vi "mod_Decimating FIR.vi"(5 "reset":bool, 6 "error in (no error)":errorcluster, 7 "taps":dbl[](array[numeric]), 8 "decimation":i32, 9 "x":dbl[](array[numeric])) -> (0 "error out":errorcluster, 3 "filtered x":dbl[](array[numeric]))   [LabVIEW 2020, in "niAMT.lvlib"]
uses:
  <vilib>/addons/Modulation/niAMT.lvlib
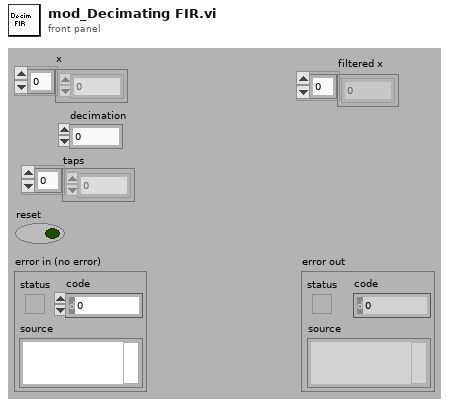
[diagram p1: front panel]
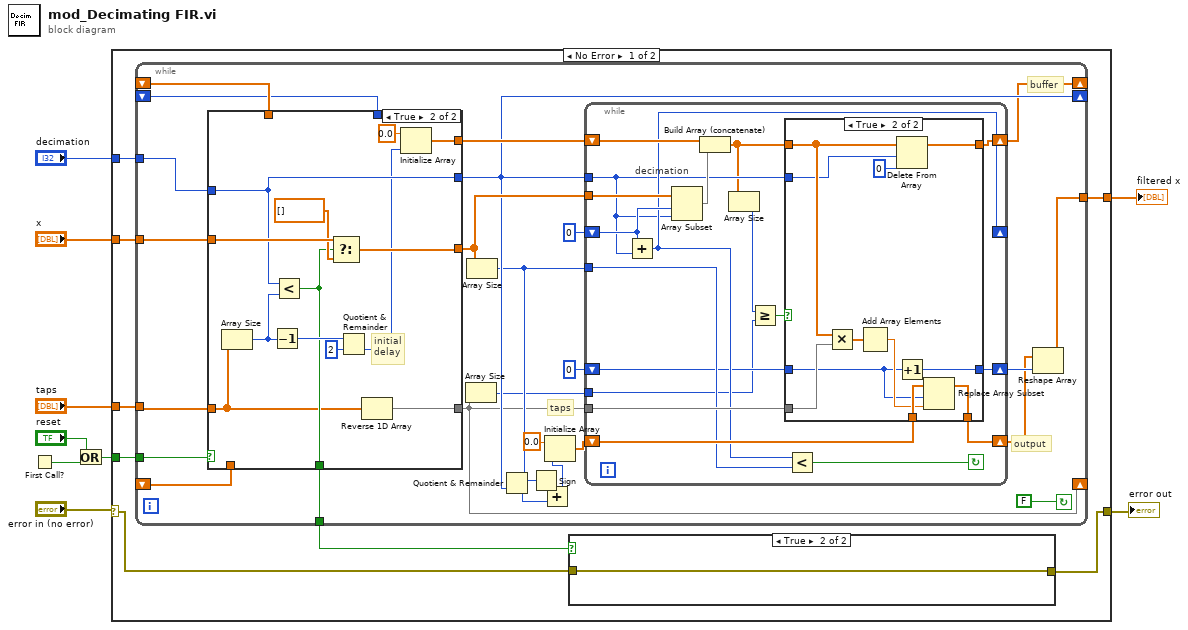
[diagram p0: block diagram]
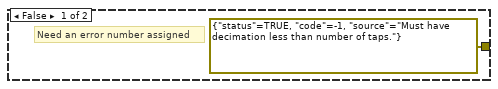
[diagram p2: hidden frame]
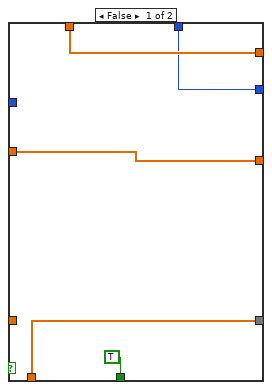
[diagram p4: hidden frame]
diagram:
  n1 = First Call?() -> (First Call?: T/F=w9:bool)
  n2 = Or(x="reset", y=w9) -> (x .or. y?=w5:bool)
  n3 = case shown="No Error" "error in (no error)" {
    selector: "error in (no error)" -> [w11 w98]
    tunnel: "x" -> [w17 w97]
    tunnel: "decimation" -> [w16 _]
    tunnel: "taps" -> [w15 _]
    tunnel: w5 -> [w14 _]
    tunnel: [w10 w98] -> w2
    tunnel: [w13 w97] -> w1
    frame No Error {
      n4 = while {
        tunnel: w14 -> [w45]
        tunnel: w17 -> [w42]
        tunnel: w16 -> [w43]
        tunnel: w15 -> [w24]
        shift-right: [w20] -> _
        shift-left: _ -> [w44]
        shift-right: [w21] -> _
        shift-left: _ -> [w41]
        tunnel: [w29] -> w13
        shift-right: [w26] -> _
        shift-left: _ -> [w40]
        tunnel: [w39] -> w12
        stop <- FALSE continue-if-true
        # "taps"
        # "output"
        # "buffer"
        n5 = case shown="True" w45 {
          tunnel: w24 -> [_ w85]
          tunnel: [w83 w96] -> w20
          tunnel: w44 -> [w83 _]
          tunnel: w43 -> [_ w87]
          tunnel: w42 -> [w82 w92]
          tunnel: [w82 w91] -> w38
          tunnel: [w81 w93] -> w27
          tunnel: w41 -> [w81 _]
          tunnel: [w80 w87] -> w26
          tunnel: w40 -> [w80 _]
          tunnel: [TRUE w89] -> w39
          frame False {
          }
          frame True {
            # "initial\ndelay"
            n6 = Array Size(array=w85) -> (size(s)=w84:i32)
            n7 = Decrement(x=w84) -> (x-1=w94:i32)
            n8 = Less?(x=w87, y=w84) -> (x < y?=w89:bool)
            n9 = Select(t=w92, s=w89, f=dbl[] []) -> (s? t:f=w91:dbl[])
            n10 = Quotient & Remainder(x=w94, y=2) -> (floor(x/y)=w86:i32)  [unwired: 1 out]
            n11 = Reverse 1D Array(array=w85) -> (reversed array=w96:dbl[])
            n12 = Initialize Array(0.0 ("element"), w86) -> (w93:dbl[])
          }
        }
        n13 = Array Size(array=w20) -> (size(s)=w23:i32)
        n14 = Array Size(array=w38) -> (size(s)=w25:i32)
        n15 = Quotient & Remainder(x=w25, y=w26) -> (x-y*floor(x/y)=w33:i32, floor(x/y)=w31:i32)
        n16 = Sign(1:w33) -> (0:w32:i32)
        n17 = Add(x=w32, y=w31) -> (x+y=w30:i32)
        n18 = Initialize Array(0.0, w30) -> (w35:dbl[])
        n19 = while {
          tunnel: w38 -> [w60]
          shift-right: [w54] -> w21
          shift-left: w27 -> [w64]
          tunnel: w20 -> [w63]
          shift-right: [w61] -> w22
          shift-left: w35 -> [w62]
          tunnel: w26 -> [w50]
          shift-right: [w57] -> _
          shift-left: 0 -> [w58]
          tunnel: w25 -> [w56]
          shift-right: [w52] -> w28
          shift-left: 0 -> [w53]
          tunnel: w23 -> [w47]
          stop <- w55 continue-if-true
          # "decimation"
          n20 = Add(x=w58, y=w50) -> (x+y=w57:i32)
          n21 = Array Subset(array=w60, index=w58, length=w50) -> (w51:dbl[])
          n22 = Build Array (concatenate)(w64, w51) -> (w49:dbl[])
          n23 = Array Size(array=w49) -> (size(s)=w48:i32)
          n24 = Greater Or Equal?(x=w48, y=w47) -> (x >= y?=w59:bool)
          n25 = case shown="True" w59 {
            tunnel: w49 -> [w67 w74]
            tunnel: w63 -> [_ w78]
            tunnel: w62 -> [w66 w77]
            tunnel: [w66 w76] -> w61
            tunnel: [w67 w73] -> w54
            tunnel: w50 -> [_ w68]
            tunnel: w53 -> [w65 w69]
            tunnel: [w65 w70] -> w52
            frame False {
            }
            frame True {
              n26 = Multiply(x=w74, y=w78) -> (x*y=w75:dbl[])
              n27 = Add Array Elements(numeric array=w75) -> (sum=w71:dbl)
              n28 = Delete From Array(array=w74, length=w68, index=0) -> (array with subset deleted=w73:dbl[])  [unwired: 1 out]
              n29 = Increment(x=w69) -> (x+1=w70:i32)
              n30 = Replace Array Subset(array=w77, new element=w71, index=w69) -> (w76:dbl[])
            }
          }
          n31 = Less?(x=w57, y=w56) -> (x < y?=w55:bool)
        }
        n32 = Reshape Array(w22, w28) -> (w29:dbl[])
      }
      n33 = case shown="True" w12 {
        tunnel: w11 -> [_ w19]
        tunnel: [errorcluster {"status"=TRUE, "code"=-1, "source"="Must have decimation less than number of taps."} ("error IO") w19] -> w10
        frame False {
          # "Need an error number assigned"
        }
        frame True {
        }
      }
    }
    frame Error {
    }
  }
  "filtered x" <- w1
  "error out" <- w2
